vi "LS Data Loop.vi"(11 "FPGA Ref":T1) -> ()   [LabVIEW 2019]
uses:
  Controls/FPGA_Reference.ctl
  <vilib>/Utility/error.llb/Error Cluster From Error Code.vi
  <vilib>/rvi/errors/niLvFpgaAdjustHostInterfaceError.vi
  <vilib>/rvi/interface/nirviMethod/nirviMethod.xnode
  FPGA Bitfiles/LS_Durability_FPGA_9627.lvbitx
  <vilib>/rvi/interface/nirviReadWriteControl/nirviReadWriteControl.xnode
  <vilib>/rvi/errors/niLvFpgaMergeErrorWithErrorCode.vi
  <vilib>/FPGAPlugInAG/sbRIO-9627/niLvFpga_ReadFifo_sbRIO-9627.vi
  NiFpgaLv.dll
panel:
  out "FIFO loops":i32
  in  "LoopWait(ms)":u32=100
  in  "Sections":i32=100
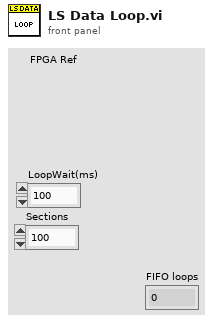
[diagram p1: front panel]
types:
  T1 = typedef "FPGA_Reference.ctl" = refnum<k20>
  T2 = cluster{"FPGA Ref":T1, "Time":dbl, "PtsTaken":i32, "Pts/File":i32, "10AveWait":u32, "Stored Filepath":path, "FileIndex":i32, "FilesUsed":i32, "Day":i32, "Anomaly Path":path}
  T3 = enum16{"Read", "Engine Writes", "Main Writes", "Write Anomalies", "Write Init Data"}
  T4 = enum16{"open", "replace", "create", "open or create", "replace or create", "replace or create with confirmation"}
  T5 = typedef "LS Data.ctl" = cluster{"Total Cycles":u32[], "Steps":u32[], "Anomalies Total":i32[], "Cycles":u32[], "Anomalies/Cycle":i32[], "Anomalies (Last Cycle)":i32[], "Opens":i32[]}
  T6 = cluster{"Running?":bool, "Profile Record":bool, "RecordInterval":i32, "RecordDuration":i32, "RecordFreq":i32, "Data Filepath":path, "Hr Record":bool, "Serial Numbers":string[]}
  T7 = typedef "LVDateTimeRec.ctl" = cluster{"fractional second":dbl, "second":i32, "minute":i32, "hour":i32, "day of month":i32, "month":i32, "year":i32, "day of week":i32, "day of year":i32, "DST":i32}
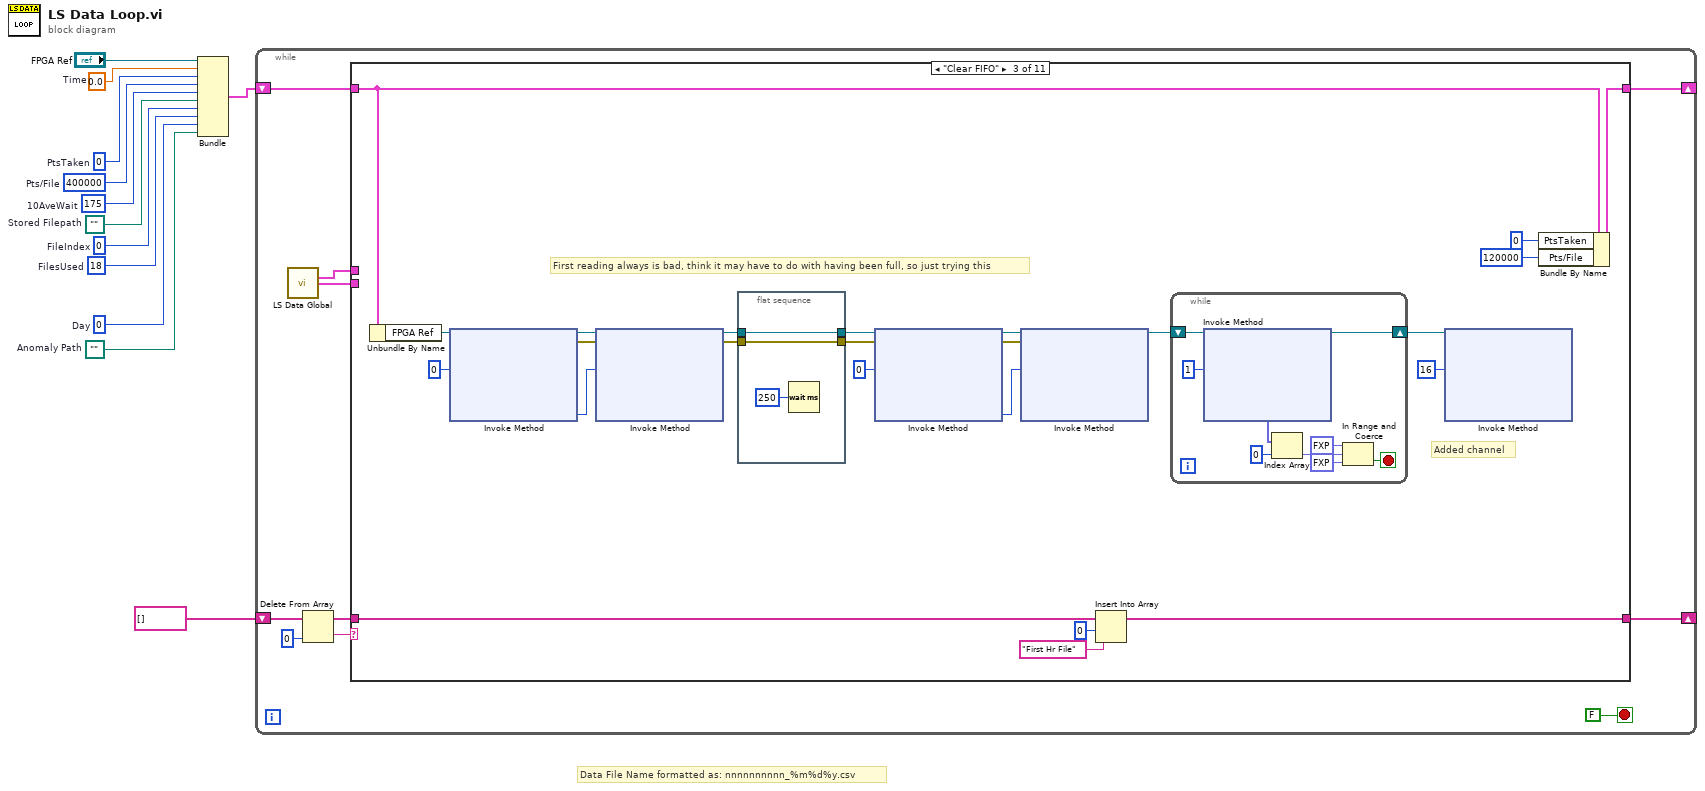
[diagram p0: block diagram]
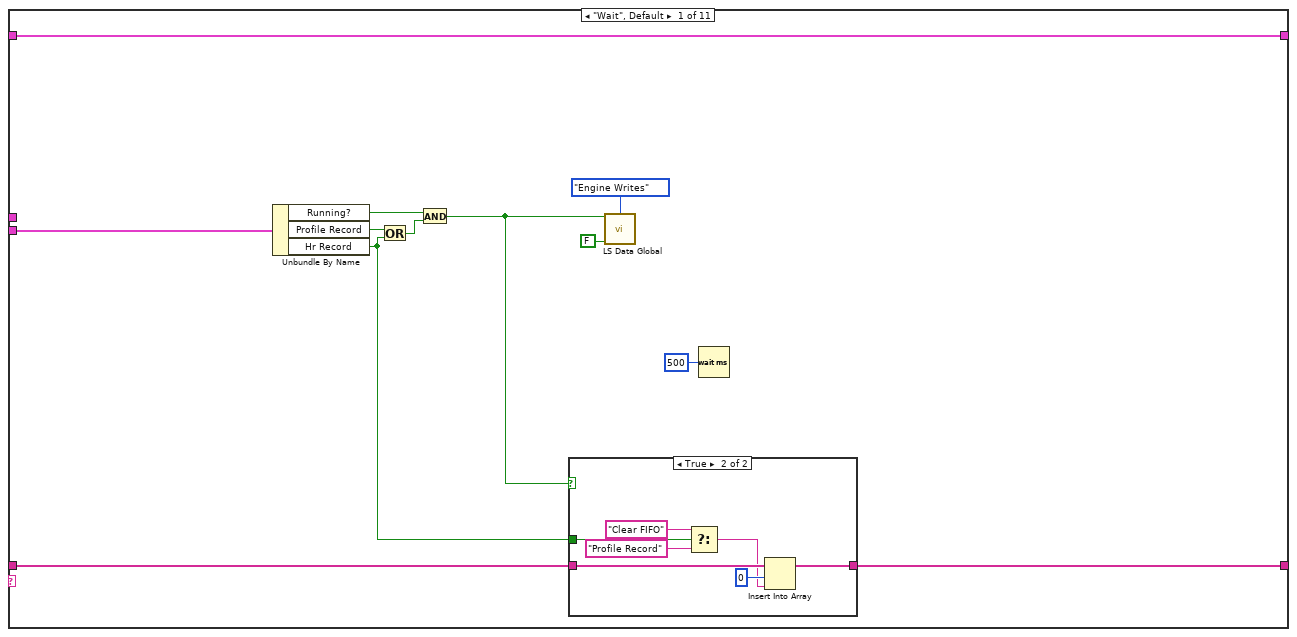
[diagram p2: hidden frame]
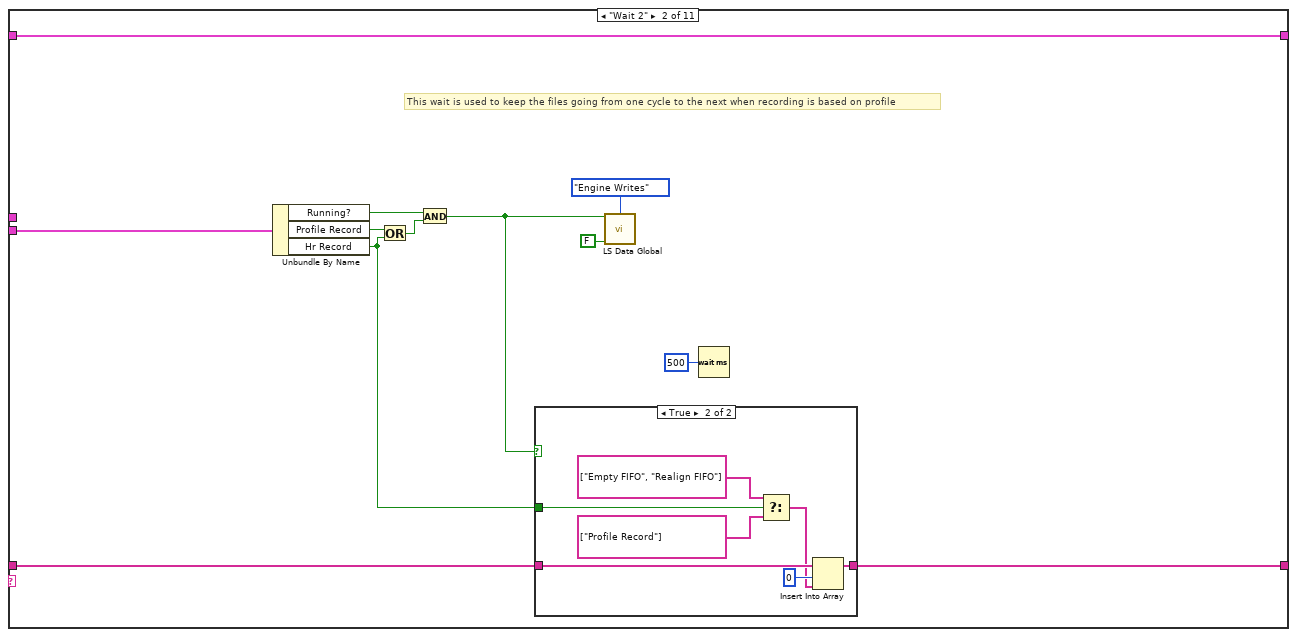
[diagram p4: hidden frame]
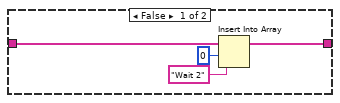
[diagram p5: hidden frame]
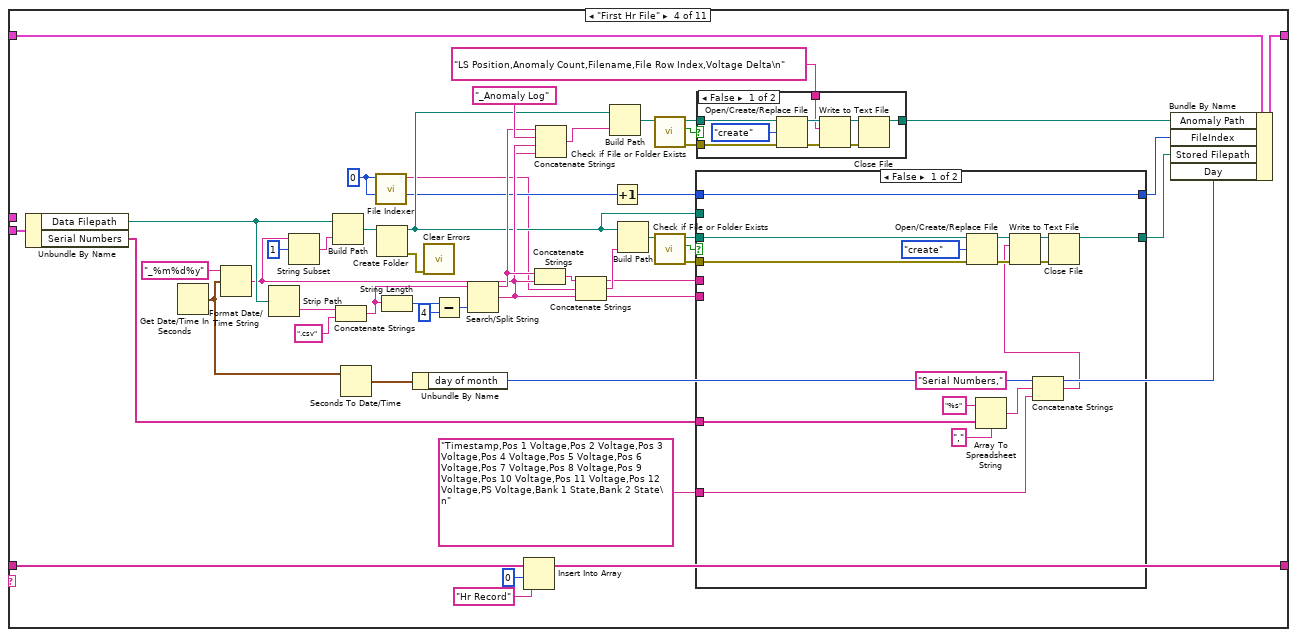
[diagram p6: hidden frame]
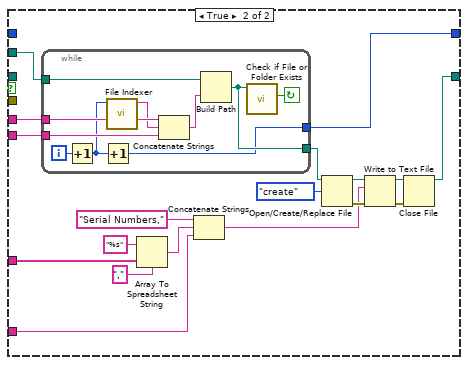
[diagram p8: hidden frame]
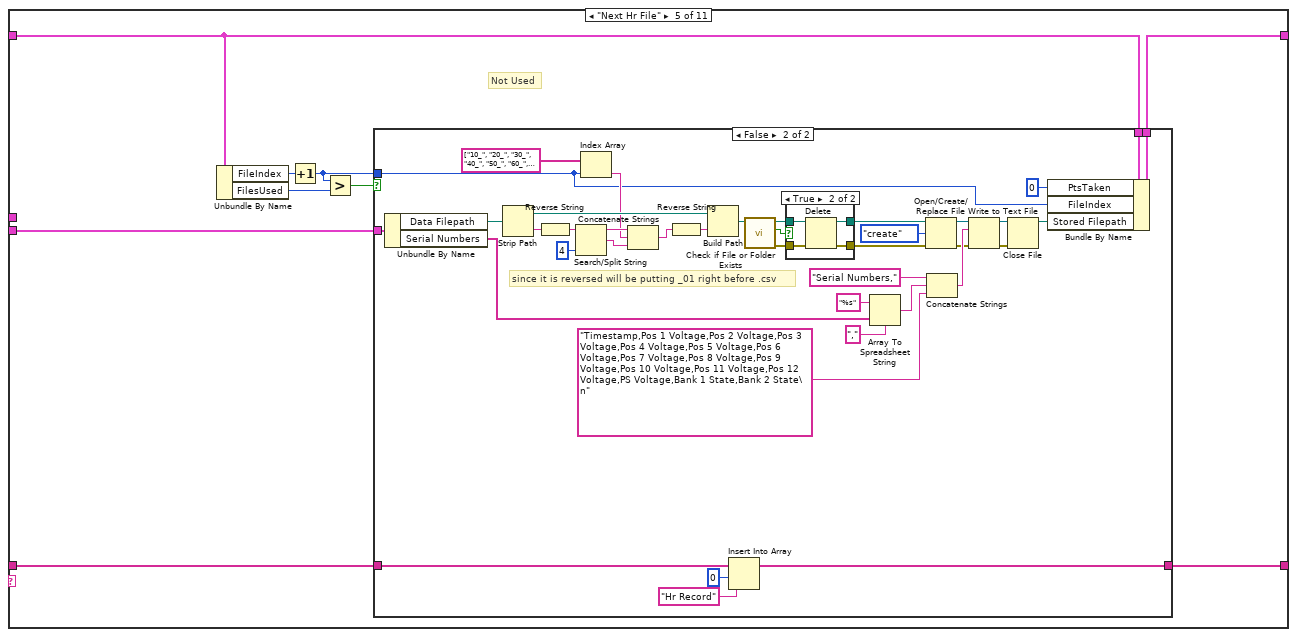
[diagram p9: hidden frame]
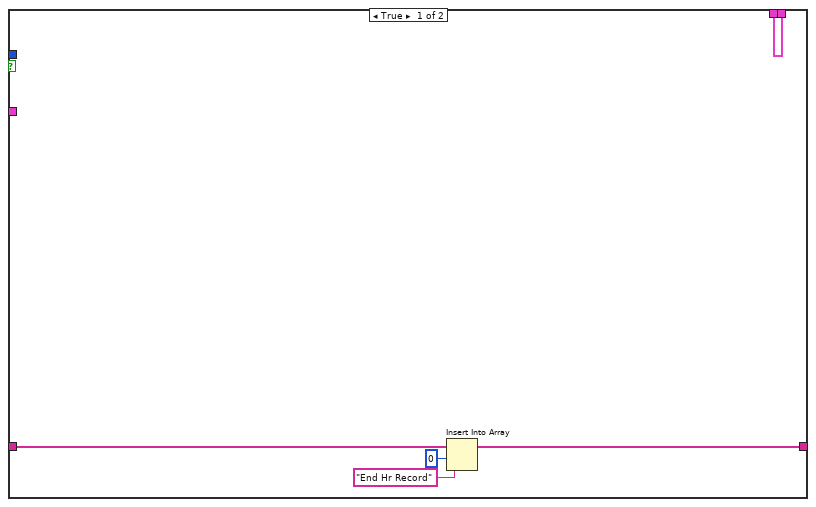
[diagram p10: hidden frame]
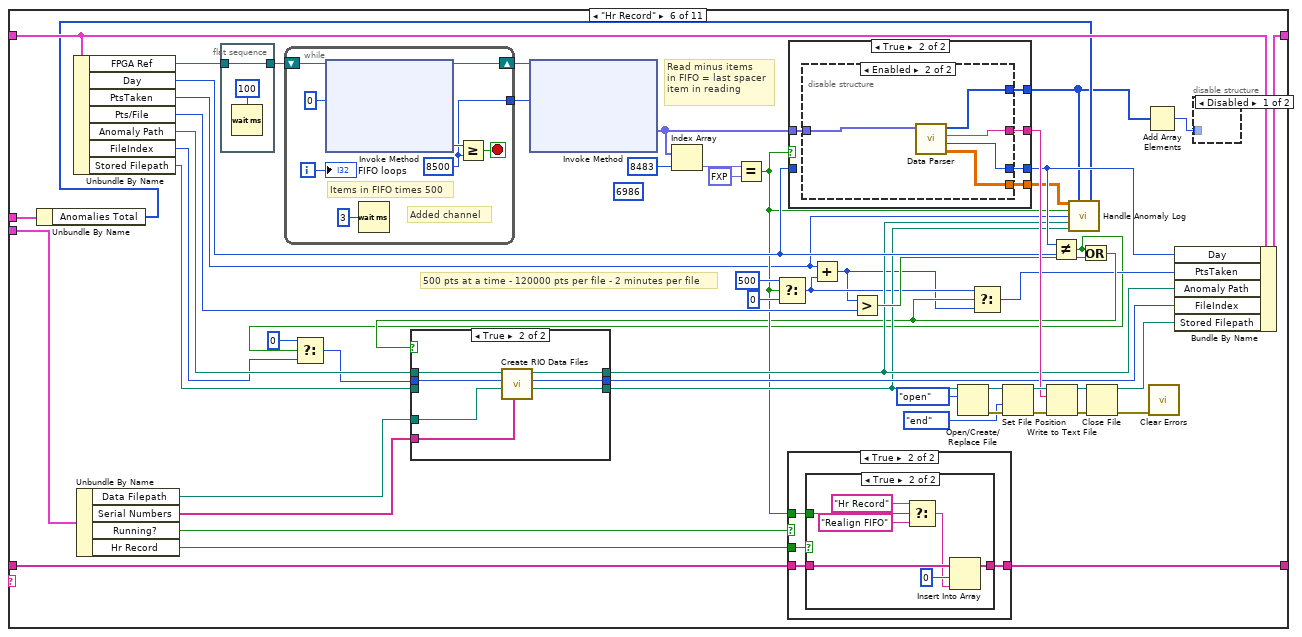
[diagram p12: hidden frame]
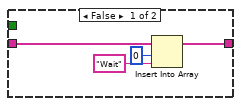
[diagram p14: hidden frame]
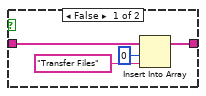
[diagram p15: hidden frame]
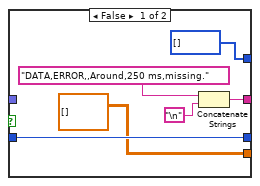
[diagram p17: hidden frame]
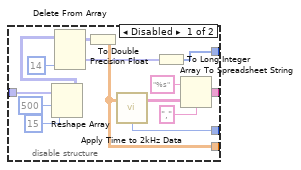
[diagram p18: hidden frame]
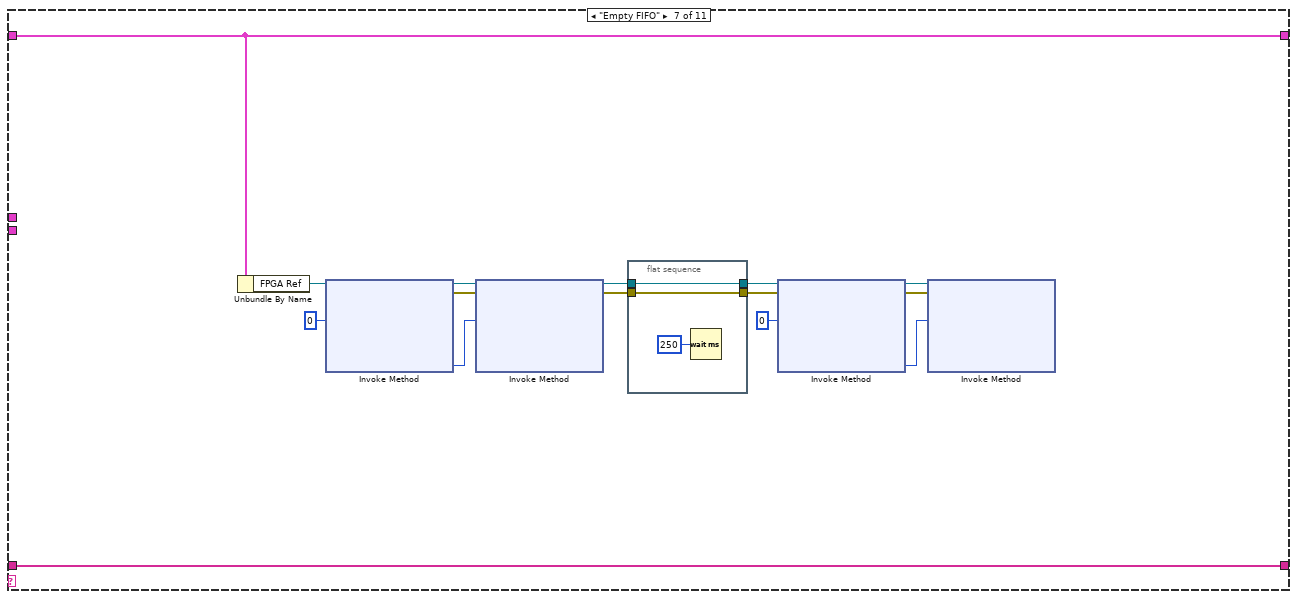
[diagram p19: hidden frame]
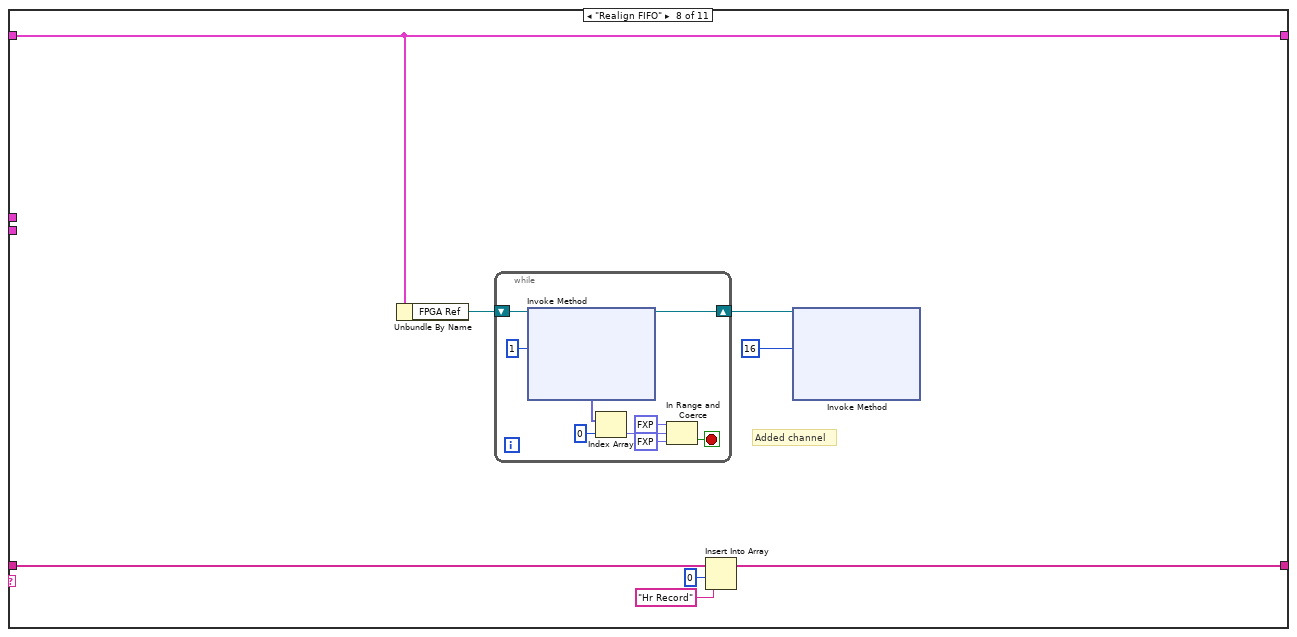
[diagram p20: hidden frame]
diagram:
  w1 = path ""  # Anomaly Path
  w2 = 0  # Day
  w3 = 18  # FilesUsed
  w4 = 0  # FileIndex
  w5 = path ""  # Stored Filepath
  w6 = u32 175  # 10AveWait
  w7 = 400000  # Pts/File
  w8 = 0  # PtsTaken
  w11 = 0.0  # Time
  # "Data File Name formatted as: nnnnnnnnnn_%m%d%y.csv"
  n1 = Bundle("FPGA Ref"="FPGA Ref", "Time"=w11, "PtsTaken"=w8, "Pts/File"=w7, "10AveWait"=w6, "Stored Filepath"=w5, "FileIndex"=w4, "FilesUsed"=w3, "Day"=w2, "Anomaly Path"=w1) -> (w10:T2)  [unwired: 1 in]
  n2 = while {
    shift-right: [w20] -> _
    shift-left: w10 -> [w21]
    shift-right: [w17] -> _
    shift-left: string[] [] -> [w19]
    stop <- FALSE stop-if-true
    n3 = call "LS Data Global.vi"() -> ("Initial LS Data Out"=w13:T5, "LS Cluster Out"=w18:T6)  [unwired: 12 in, 2 out]
    n4 = Delete From Array(array=w19, index=0) -> (deleted portion=w15:string, array with subset deleted=w14:string[])  [unwired: 1 in]
    n5 = case shown="\"Clear FIFO\"" w15 {
      tunnel: w14 -> [w31 w51 w85 w146 w203 w277 w398 w404 w428 w437 w440]
      tunnel: [w30 w50 w83 w145 w209 w276 w398 w403 w427 w436 w439] -> w17
      tunnel: w18 -> [w32 w52 _ w148 w211 w315 _ _ _ _ w441]
      tunnel: w21 -> [w29 w49 w81 w142 w208 w298 w399 w407 w424 w438 w443]
      tunnel: [w29 w49 w80 w147 w210 w297 w399 w407 w424 w438 w442] -> w20
      tunnel: w13 -> [_ _ _ _ _ w265 _ _ _ _ _]
      frame "Wait", Default {
        n6 = Unbundle By Name(w32) -> ("Running?"=w33:bool, "Profile Record"=w28:bool, "Hr Record"=w26:bool)
        n7 = Or(x=w28, y=w26) -> (x .or. y?=w27:bool)
        n8 = And(x=w33, y=w27) -> (x .and. y?=w25:bool)
        n9 = case shown="True" w25 {
          tunnel: w31 -> [w35 w42]
          tunnel: [w35 w41] -> w30
          tunnel: w26 -> [_ w39]
          frame False {
          }
          frame True {
            n10 = Select(t="Clear FIFO" ("new element/subarray"), s=w39, f="Profile Record" ("new element/subarray")) -> (s? t:f=w37:string)
            n11 = Insert Into Array(array=w42, index=0, new element=w37) -> (w41:string[])
          }
        }
        n12 = call "LS Data Global.vi"("Recording In"=w25, "Mode"=T3."Engine Writes", "Transferring In"=FALSE) -> ()  [unwired: 9 in, 4 out]
        n13 = Wait (ms)(milliseconds to wait=u32 500) -> ()  [unwired: 1 out]
      }
      frame "Wait 2" {
        # "This wait is used to keep the files going from one cycle to the next when recording is based on profile"
        n14 = Unbundle By Name(w52) -> ("Running?"=w53:bool, "Profile Record"=w48:bool, "Hr Record"=w46:bool)
        n15 = Or(x=w48, y=w46) -> (x .or. y?=w47:bool)
        n16 = And(x=w53, y=w47) -> (x .and. y?=w45:bool)
        n17 = case shown="True" w45 {
          tunnel: w51 -> [w58 w65]
          tunnel: [w57 w64] -> w50
          tunnel: w46 -> [_ w62]
          frame False {
            n18 = Insert Into Array(array=w58, index=0, new element="Wait 2" ("new element/subarray")) -> (w57:string[])
          }
          frame True {
            n19 = Select(t=string[] ["Empty FIFO", "Realign FIFO"], s=w62, f=string[] ["Profile Record"]) -> (s? t:f=w61:string[])
            n20 = Insert Into Array(array=w65, index=0, new element=w61) -> (w64:string[])
          }
        }
        n21 = call "LS Data Global.vi"("Recording In"=w45, "Mode"=T3."Engine Writes", "Transferring In"=FALSE) -> ()  [unwired: 9 in, 4 out]
        n22 = Wait (ms)(milliseconds to wait=u32 500) -> ()  [unwired: 1 out]
      }
      frame "Clear FIFO" {
        # "First reading always is bad, think it may have to do with having been full, so just trying this"
        # "Added channel"
        n23 = Unbundle By Name(w81) -> ("FPGA Ref"=w66:T1)
        n24 = xnode "Invoke Method"("FPGA VI Reference In"=w66, "Number of Elements"=u32 0) -> ("FPGA VI Reference Out"=w89:T1, "error out"=w88:errorcluster, "Elements Remaining"=w86:u32)  [unwired: 2 in, 1 out]
        n25 = xnode "Invoke Method"("FPGA VI Reference In"=w89, "error in"=w88, "Number of Elements"=w86) -> ("FPGA VI Reference Out"=w70:T1, "error out"=w69:errorcluster)  [unwired: 1 in, 2 out]
        n26 = flat-sequence {
          tunnel: w70 -> [w92]
          tunnel: w69 -> [w91]
          tunnel: [w92] -> w68
          tunnel: [w91] -> w67
          frame #0 {
            n27 = Wait (ms)(milliseconds to wait=u32 250) -> ()  [unwired: 1 out]
          }
        }
        n28 = xnode "Invoke Method"("FPGA VI Reference In"=w68, "error in"=w67, "Number of Elements"=u32 0) -> ("FPGA VI Reference Out"=w72:T1, "error out"=w73:errorcluster, "Elements Remaining"=w75:u32)  [unwired: 1 in, 1 out]
        n29 = xnode "Invoke Method"("FPGA VI Reference In"=w72, "error in"=w73, "Number of Elements"=w75) -> ("FPGA VI Reference Out"=w71:T1)  [unwired: 1 in, 3 out]
        n30 = Insert Into Array(array=w85, index=0, new element="First Hr File" ("new element/subarray")) -> (w83:string[])
        n31 = while {
          shift-right: [w100] -> w76
          shift-left: w71 -> [w101]
          stop <- w93 stop-if-true
          n32 = xnode "Invoke Method"("FPGA VI Reference In"=w101, "Number of Elements"=u32 1) -> ("FPGA VI Reference Out"=w100:T1, "Data"=w98:fxp<+/-,22,11>[])  [unwired: 2 in, 2 out]
          n33 = Index Array(array=w98, index=0) -> (element=w96:fxp<+/-,22,11>)
          n34 = In Range and Coerce(upper limit=fxp<+/-,18,5> -14.0, x=w96, lower limit=fxp<+/-,18,5> -15.0) -> (In Range?=w93:bool)  [unwired: 1 out]
        }
        n35 = xnode "Invoke Method"("FPGA VI Reference In"=w76, "Number of Elements"=u32 16) -> ()  [unwired: 2 in, 4 out]
        n36 = Bundle By Name(cluster=w81, "PtsTaken"=0, "Pts/File"=120000 ("PtsNeeded")) -> (w80:T2)
      }
      frame "First Hr File" {
        w104 = 0
        n37 = Unbundle By Name(w148) -> ("Data Filepath"=w127:path, "Serial Numbers"=w116:string[])
        n38 = Get Date/Time In Seconds() -> (seconds since 1Jan1904=w106:timestamp)
        n39 = Format Date/Time String(time format string (%c)="_%m%d%y", seconds (now)=w106) -> (date/time string=w112:string)  [unwired: 1 in]
        n40 = Strip Path(path=w127) -> (name=w139:string)  [unwired: 1 out]
        n41 = String Subset(string=w112, offset (0)=1) -> (substring=w137:string)  [unwired: 1 in]
        n42 = Build Path(base path=w127, name or relative path=w137) -> (appended path=w125:path)
        n43 = Concatenate Strings(w139, ".csv" ("string")) -> (w141:string)
        n44 = Seconds To Date/Time(time stamp (now)=w106) -> (date time rec=w107:T7)  [unwired: 1 in]
        n45 = call "File Indexer.vi"("File Index In"=w104) -> ("File Indicator Out"=w103:string)  [unwired: 10 in]
        n46 = Create Folder(path (use dialog)=w125) -> (created path=w108:path, error out=w126:errorcluster)  [unwired: 2 in, 1 out]
        n47 = String Length(string=w141) -> (length=w133:i32)
        n48 = Unbundle By Name(w107) -> ("day of month"=w105:i32)
        n49 = call <vilib>:"Clear Errors.vi"("error in (no error)"=w126) -> ()  [unwired: 5 in, 2 out]
        n50 = Subtract(x=w133, y=4) -> (x-y=w135:i32)
        n51 = Search/Split String(string=w141, offset (0)=w135) -> (substring before match=w113:string, match + rest of string=w109:string)  [unwired: 1 in, 1 out]
        n52 = Insert Into Array(array=w146, index=0, new element="Hr Record" ("new element/subarray")) -> (w145:string[])
        n53 = Concatenate Strings(w113, w112) -> (w110:string)
        n54 = Concatenate Strings(w113, "_Anomaly Log" ("string"), w112, w109) -> (w123:string)
        n55 = Concatenate Strings(w110, w103, w109) -> (w111:string)
        n56 = Build Path(base path=w108, name or relative path=w123) -> (appended path=w121:path)
        n57 = Increment(x=w104) -> (x+1=w115:i32)
        n58 = Build Path(base path=w108, name or relative path=w111) -> (appended path=w132:path)
        n59 = call <vilib>:"Check if File or Folder Exists.vi"("path"=w121) -> ("error out"=w118:errorcluster, "file or folder exists?"=w120:bool, "dup path"=w119:path)  [unwired: 8 in]
        n60 = call <vilib>:"Check if File or Folder Exists.vi"("path"=w132) -> ("error out"=w129:errorcluster, "file or folder exists?"=w131:bool, "dup path"=w130:path)  [unwired: 8 in]
        n61 = case shown="False" w131 {
          tunnel: w130 -> [w169 _]
          tunnel: [w168 w177] -> w124
          tunnel: w129 -> [w167 _]
          tunnel: w116 -> [w162 w184]
          tunnel: w115 -> [w160 _]
          tunnel: [w160 w189] -> w114
          tunnel: w110 -> [_ w191]
          tunnel: w109 -> [_ w190]
          tunnel: w108 -> [_ w192]
          tunnel: "Timestamp,Pos 1 Voltage,Pos 2 Voltage,Pos 3 Voltage,Pos 4 Voltage,Pos 5 Voltage,Pos 6 Voltage,Pos 7 Voltage,Pos 8 Voltage,Pos 9 Voltage,Pos 10 Voltage,Pos 11 Voltage,Pos 12 Voltage,PS Voltage,Bank 1 State,Bank 2 State\n" -> [w159 w175]
          frame False {
            n62 = Open/Create/Replace File(file path (use dialog)=w169, error in=w167, operation (0:open)=T4."create") -> (refnum out=w171:refnum<file>, error out=w173:errorcluster)  [unwired: 3 in, 1 out]
            n63 = Array To Spreadsheet String(delimiter (Tab)=",", array=w162, 3:"%s" ("format string")) -> (spreadsheet string=w163:string)
            n64 = Concatenate Strings("Serial Numbers," ("string"), w163, w159) -> (w161:string)
            n65 = Write to Text File(file (use dialog)=w171, text=w161, error in=w173) -> (refnum out=w170:refnum<file>, error out=w172:errorcluster)  [unwired: 1 in, 1 out]
            n66 = Close File(refnum=w170, error in=w172) -> (path=w168:path)  [unwired: 1 out]
          }
          frame True {
            n67 = while {
              tunnel: w192 -> [w202]
              tunnel: w191 -> [w201]
              tunnel: w190 -> [w200]
              tunnel: [w197] -> w178
              tunnel: [w195] -> w189
              i -> [w196]
              stop <- w198 continue-if-true
              n68 = Increment(x=w196) -> (x+1=w194:i32)
              n69 = Increment(x=w194) -> (x+1=w195:i32)
              n70 = call "File Indexer.vi"("File Index In"=w194) -> ("File Indicator Out"=w193:string)  [unwired: 10 in]
              n71 = Concatenate Strings(w201, w193, w200) -> (w199:string)
              n72 = Build Path(base path=w202, name or relative path=w199) -> (appended path=w197:path)
              n73 = call <vilib>:"Check if File or Folder Exists.vi"("path"=w197) -> ("file or folder exists?"=w198:bool)  [unwired: 8 in, 2 out]
            }
            n74 = Array To Spreadsheet String(delimiter (Tab)=",", array=w184, 3:"%s" ("format string")) -> (spreadsheet string=w185:string)
            n75 = Concatenate Strings("Serial Numbers," ("string"), w185, w175) -> (w176:string)
            n76 = Open/Create/Replace File(file path (use dialog)=w178, operation (0:open)=T4."create") -> (refnum out=w180:refnum<file>, error out=w182:errorcluster)  [unwired: 4 in, 1 out]
            n77 = Write to Text File(file (use dialog)=w180, text=w176, error in=w182) -> (refnum out=w179:refnum<file>, error out=w181:errorcluster)  [unwired: 1 in, 1 out]
            n78 = Close File(refnum=w179, error in=w181) -> (path=w177:path)  [unwired: 1 out]
          }
        }
        n79 = case shown="False" w120 {
          tunnel: w119 -> [w151 w158]
          tunnel: [w152 w158] -> w128
          tunnel: w118 -> [w150 _]
          tunnel: "LS Position,Anomaly Count,Filename,File Row Index,Voltage Delta\n" -> [w149 _]
          frame False {
            n80 = Open/Create/Replace File(file path (use dialog)=w151, error in=w150, operation (0:open)=T4."create") -> (refnum out=w154:refnum<file>, error out=w156:errorcluster)  [unwired: 3 in, 1 out]
            n81 = Write to Text File(file (use dialog)=w154, text=w149, error in=w156) -> (refnum out=w153:refnum<file>, error out=w155:errorcluster)  [unwired: 1 in, 1 out]
            n82 = Close File(refnum=w153, error in=w155) -> (path=w152:path)  [unwired: 1 out]
          }
          frame True {
          }
        }
        n83 = Bundle By Name(cluster=w142, "Anomaly Path"=w128, "FileIndex"=w114, "Stored Filepath"=w124, "Day"=w105) -> (w147:T2)
      }
      frame "Next Hr File" {
        # "Not Used"
        n84 = Unbundle By Name(w208) -> ("FileIndex"=w207:i32, "FilesUsed"=w206:i32)
        n85 = Increment(x=w207) -> (x+1=w205:i32)
        n86 = Greater?(x=w205, y=w206) -> (0:w204:bool)
        n87 = case shown="False" w204 {
          tunnel: w211 -> [_ w255]
          tunnel: [w216 w254] -> w210
          tunnel: [w214 w243] -> w209
          tunnel: w208 -> [w216 w222]
          tunnel: w205 -> [_ w220]
          tunnel: w203 -> [w215 w244]
          frame True {
            n88 = Insert Into Array(array=w215, index=0, new element="End Hr Record" ("new element/subarray")) -> (w214:string[])
          }
          frame False {
            # "since it is reversed will be putting _01 right before .csv"
            n89 = Unbundle By Name(w255) -> ("Data Filepath"=w253:path, "Serial Numbers"=w223:string[])
            n90 = Strip Path(path=w253) -> (stripped path=w252:path, name=w251:string)
            n91 = Reverse String(1:w251) -> (0:w249:string)
            n92 = Search/Split String(string=w249, offset (0)=4) -> (substring before match=w247:string, match + rest of string=w245:string)  [unwired: 1 in, 1 out]
            n93 = Index Array(array=string[] ["10_", "20_", "30_", "40_", "50_", "60_", "70_", "80_", "90_", "01_", "11_", "21_", "31_", "41_", "51_", "61_", "71_", "81_", "91_", "02_", "12_", "22_", "32_", "42_", "52_", "62_", "72_", "82_", "92_", "03_", "13_", "23_", "33_", "43_", "53_", "63_", "73_", "83_", "93_", "04_", "14_", "24_", "34_", "44_", "54_", "64_", "74_", "84_", "94_", "05_", "15_", "25_", "35_", "45_", "55_", "65_", "75_", "85_", "95_", "06_", "16_", "26_", "36_", "46_", "56_", "66_", "76_", "86_", "96_", "07_", "17_", "27_", "37_", "47_", "57_", "67_", "77_", "87_", "97_", "08_", "18_", "28_", "38_", "48_", "58_", "68_", "78_", "88_", "98_", "09_", "19_", "29_", "39_", "49_", "59_", "69_", "79_", "89_", "99_"] ("Array 2"), index=w220) -> (element=w221:string)
            n94 = Concatenate Strings(w247, w221, w245) -> (w246:string)
            n95 = Reverse String(1:w246) -> (0:w250:string)
            n96 = Build Path(base path=w252, name or relative path=w250) -> (appended path=w240:path)
            n97 = Insert Into Array(array=w244, index=0, new element="Hr Record" ("new element/subarray")) -> (w243:string[])
            n98 = call <vilib>:"Check if File or Folder Exists.vi"("path"=w240) -> ("error out"=w225:errorcluster, "file or folder exists?"=w239:bool, "dup path"=w238:path)  [unwired: 8 in]
            n99 = case shown="True" w239 {
              tunnel: w238 -> [w257 w261]
              tunnel: [w257 w260] -> w227
              tunnel: w225 -> [w256 w259]
              tunnel: [w256 w258] -> w224
              frame False {
              }
              frame True {
                n100 = Delete(path (use dialog)=w261, error in=w259) -> (deleted path=w260:path, error out=w258:errorcluster)  [unwired: 3 in, 1 out]
              }
            }
            n101 = Array To Spreadsheet String(delimiter (Tab)=",", array=w223, 3:"%s" ("format string")) -> (spreadsheet string=w237:string)
            n102 = Open/Create/Replace File(file path (use dialog)=w227, error in=w224, operation (0:open)=T4."create") -> (refnum out=w231:refnum<file>, error out=w229:errorcluster)  [unwired: 3 in, 1 out]
            n103 = Concatenate Strings("Serial Numbers," ("string"), w237, "Timestamp,Pos 1 Voltage,Pos 2 Voltage,Pos 3 Voltage,Pos 4 Voltage,Pos 5 Voltage,Pos 6 Voltage,Pos 7 Voltage,Pos 8 Voltage,Pos 9 Voltage,Pos 10 Voltage,Pos 11 Voltage,Pos 12 Voltage,PS Voltage,Bank 1 State,Bank 2 State\n") -> (w234:string)
            n104 = Write to Text File(file (use dialog)=w231, text=w234, error in=w229) -> (refnum out=w232:refnum<file>, error out=w230:errorcluster)  [unwired: 1 in, 1 out]
            n105 = Close File(refnum=w232, error in=w230) -> (path=w226:path)  [unwired: 1 out]
            n106 = Bundle By Name(cluster=w222, "PtsTaken"=0, "FileIndex"=w220, "Stored Filepath"=w226) -> (w254:T2)
          }
        }
      }
      frame "Hr Record" {
        (unwired) 6986 ("index")
        # "Read minus items\nin FIFO = last spacer\nitem in reading"
        # "500 pts at a time - 120000 pts per file - 2 minutes per file"
        n107 = Unbundle By Name(w265) -> ("Anomalies Total"=w264:i32[])
        n108 = Unbundle By Name(w298) -> ("FPGA Ref"=w303:T1, "Day"=w290:i32, "PtsTaken"=w274:i32, "Pts/File"=w296:i32, "Anomaly Path"=w288:path, "FileIndex"=w268:i32, "Stored Filepath"=w287:path)
        n109 = Unbundle By Name(w315) -> ("Data Filepath"=w275:path, "Serial Numbers"=w284:string[], "Running?"=w279:bool, "Hr Record"=w278:bool)
        n110 = flat-sequence {
          tunnel: w303 -> [w376]
          tunnel: [w376] -> w302
          frame #0 {
            n111 = Wait (ms)(milliseconds to wait=u32 100) -> ()  [unwired: 1 out]
          }
        }
        n112 = while {
          tunnel: [w382] -> w314
          shift-right: [w379] -> w313
          shift-left: w302 -> [w380]
          i -> [w378]
          stop <- w381 stop-if-true
          w382 = u32 8500 ("y")
          # "Added channel"
          # "Items in FIFO times 500"
          n113 = xnode "Invoke Method"("FPGA VI Reference In"=w380, "Number of Elements"=u32 0) -> ("FPGA VI Reference Out"=w379:T1, "Elements Remaining"=w383:u32)  [unwired: 2 in, 2 out]
          n114 = Wait (ms)(milliseconds to wait=u32 3) -> ()  [unwired: 1 out]
          n115 = Greater Or Equal?(x=w383, y=w382) -> (x >= y?=w381:bool)
          "FIFO loops" <- w378
        }
        n116 = xnode "Invoke Method"("FPGA VI Reference In"=w313, "Number of Elements"=w314) -> ("Data"=w295:fxp<+/-,22,11>[])  [unwired: 2 in, 3 out]
        n117 = Index Array(array=w295, index=8483) -> (element=w294:fxp<+/-,22,11>)
        n118 = Equal?(x=w294, y=fxp<+/-,18,5> -15.0) -> (x = y?=w280:bool)
        n119 = Select(t=500 ("PtsTaken"), s=w280, f=0 ("PtsTaken")) -> (s? t:f=w272:i32)
        n120 = case shown="True" w279 {
          tunnel: w277 -> [w318 w323]
          tunnel: [w317 w322] -> w276
          tunnel: w280 -> [_ w320]
          tunnel: w278 -> [_ w321]
          frame False {
            n121 = Insert Into Array(array=w318, index=0, new element="Wait") -> (w317:string[])
          }
          frame True {
            n122 = case shown="True" w321 {
              tunnel: w323 -> [w327 w334]
              tunnel: [w326 w333] -> w322
              tunnel: w320 -> [_ w331]
              frame False {
                n123 = Insert Into Array(array=w327, index=0, new element="Transfer Files") -> (w326:string[])
              }
              frame True {
                n124 = Select(t="Hr Record", s=w331, f="Realign FIFO" ("new element/subarray")) -> (s? t:f=w329:string)
                n125 = Insert Into Array(array=w334, index=0, new element=w329) -> (w333:string[])
              }
            }
          }
        }
        n126 = case shown="True" w280 {
          tunnel: [w348 w355] -> w292
          tunnel: w295 -> [_ w353]
          tunnel: [w347 w354] -> w291
          tunnel: w290 -> [w347 _]
          tunnel: [dbl[][] [] w352] -> w283
          tunnel: [i32[] [] w351] -> w263
          frame False {
            n127 = Concatenate Strings("DATA,ERROR,,Around,250 ms,missing." ("string"), "\n") -> (w348:string)
          }
          frame True {
            n128 = disable-structure shown="Enabled" {
              disable-tunnel: [w365 w372] -> w355
              disable-tunnel: [w363 w371] -> w354
              disable-tunnel: w353 -> [w362 w374]
              disable-tunnel: [w358 w370] -> w352
              disable-tunnel: [w356 w373] -> w351
              frame Disabled {
                n129 = Reshape Array(w362, 500 ("dimension size"), 15 ("dimension size")) -> (w361:fxp<+/-,22,11>[][])
                n130 = Delete From Array(array=w361, index (col)=14 ("disabled index (col)")) -> (deleted portion=w357:fxp<+/-,22,11>[], array with subset deleted=w359:fxp<+/-,22,11>[][])  [unwired: 2 in]
                n131 = To Double Precision Float(number=w359) -> (double precision float=w358:dbl[][])
                n132 = call "Apply Time to 2kHz Data.vi"("Data In"=w358) -> ("Day"=w363:i32, "Data Out"=w364:string[][])  [unwired: 2 in]
                n133 = To Long Integer(number=w357) -> (32bit integer=w356:i32[])
                n134 = Array To Spreadsheet String(delimiter (Tab)=",", array=w364, 3:"%s" ("format string")) -> (spreadsheet string=w365:string)
              }
              frame Enabled {
                n135 = call "Data Parser.vi"("Raw Data"=w374) -> ("Data Out"=w370:dbl[][], "Day"=w371:i32, "CSV String"=w372:string, "Anomaly Array"=w373:i32[])  [unwired: 7 in]
              }
            }
          }
        }
        n136 = Add(x=w274, y=w272) -> (x+y=w271:i32)
        n137 = Greater?(x=w271, y=w296) -> (0:w289:bool)
        n138 = Not Equal?(x=w291, y=w290) -> (x != y?=w269:bool)
        n139 = Select(t=0, s=w269, f=w268) -> (s? t:f=w267:i32)
        n140 = Or(x=w269, y=w289) -> (x .or. y?=w273:bool)
        n141 = case shown="True" w273 {
          tunnel: w287 -> [w337 _]
          tunnel: [w337 w344] -> w281
          tunnel: w288 -> [w336 w343]
          tunnel: [w336 w342] -> w282
          tunnel: w267 -> [w335 w341]
          tunnel: [w335 w340] -> w285
          tunnel: w284 -> [_ w339]
          tunnel: w275 -> [_ w338]
          frame False {
          }
          frame True {
            n142 = call "Create RIO Data Files.vi"("Serial Numbers"=w339, "Base Filepath"=w338, "File Index In"=w341, "Anomaly Filepath In"=w343) -> ("Current Filepath"=w344:path, "File Index Out"=w340:i32, "Anomaly Filepath Out"=w342:path)  [unwired: 5 in]
          }
        }
        n143 = Open/Create/Replace File(file path (use dialog)=w281, operation (0:open)=T4."open") -> (refnum out=w308:refnum<file>, error out=w307:errorcluster)  [unwired: 4 in, 1 out]
        n144 = Select(t=w272, s=w273, f=w271) -> (s? t:f=w270:i32)
        n145 = Set File Position(refnum=w308, from (0:start)=enum16{"start", "end", "current"}."end", error in=w307) -> (refnum out=w305:refnum<file>, error out=w304:errorcluster)  [unwired: 1 in]
        n146 = Write to Text File(file (use dialog)=w305, text=w292, error in=w304) -> (refnum out=w311:refnum<file>, error out=w312:errorcluster)  [unwired: 1 in, 1 out]
        n147 = call "Handle Anomaly Log.vi"("Data"=w283, "FPGAnomalies"=w263, "Init Anomalies"=w264, "Enable"=w280, "RowCount In"=w274, "Anomaly Log Path"=w282, "Current Data Path"=w281) -> ()  [unwired: 9 in]
        n148 = Close File(refnum=w311, error in=w312) -> (path=w286:path, error out=w310:errorcluster)
        n149 = Add Array Elements(numeric array=w263) -> (sum=w262:i32)
        n150 = call <vilib>:"Clear Errors.vi"("error in (no error)"=w310) -> ()  [unwired: 5 in, 2 out]
        n151 = Bundle By Name(cluster=w298, "Day"=w291, "PtsTaken"=w270, "Anomaly Path"=w282, "FileIndex"=w285, "Stored Filepath"=w286) -> (w297:T2)
        n152 = disable-structure shown="Disabled" {
          disable-tunnel: w262 -> [_ _]
          frame Disabled {
          }
          frame Enabled {
          }
        }
      }
      frame "Empty FIFO" {
        n153 = Unbundle By Name(w399) -> ("FPGA Ref"=w397:T1)
        n154 = xnode "Invoke Method"("FPGA VI Reference In"=w397, "Number of Elements"=u32 0) -> ("FPGA VI Reference Out"=w396:T1, "error out"=w395:errorcluster, "Elements Remaining"=w393:u32)  [unwired: 2 in, 1 out]
        n155 = xnode "Invoke Method"("FPGA VI Reference In"=w396, "error in"=w395, "Number of Elements"=w393) -> ("FPGA VI Reference Out"=w388:T1, "error out"=w387:errorcluster)  [unwired: 1 in, 2 out]
        n156 = flat-sequence {
          tunnel: w388 -> [w402]
          tunnel: w387 -> [w401]
          tunnel: [w402] -> w386
          tunnel: [w401] -> w385
          frame #0 {
            n157 = Wait (ms)(milliseconds to wait=u32 250) -> ()  [unwired: 1 out]
          }
        }
        n158 = xnode "Invoke Method"("FPGA VI Reference In"=w386, "error in"=w385, "Number of Elements"=u32 0) -> ("FPGA VI Reference Out"=w389:T1, "error out"=w390:errorcluster, "Elements Remaining"=w392:u32)  [unwired: 1 in, 1 out]
        n159 = xnode "Invoke Method"("FPGA VI Reference In"=w389, "error in"=w390, "Number of Elements"=w392) -> ()  [unwired: 1 in, 4 out]
      }
      frame "Realign FIFO" {
        # "Added channel"
        n160 = Unbundle By Name(w407) -> ("FPGA Ref"=w410:T1)
        n161 = while {
          shift-right: [w418] -> w408
          shift-left: w410 -> [w419]
          stop <- w411 stop-if-true
          n162 = xnode "Invoke Method"("FPGA VI Reference In"=w419, "Number of Elements"=u32 1) -> ("FPGA VI Reference Out"=w418:T1, "Data"=w416:fxp<+/-,22,11>[])  [unwired: 2 in, 2 out]
          n163 = Index Array(array=w416, index=0) -> (element=w414:fxp<+/-,22,11>)
          n164 = In Range and Coerce(upper limit=fxp<+/-,18,5> -14.0, x=w414, lower limit=fxp<+/-,18,5> -15.0) -> (In Range?=w411:bool)  [unwired: 1 out]
        }
        n165 = Insert Into Array(array=w404, index=0, new element="Hr Record" ("new element/subarray")) -> (w403:string[])
        n166 = xnode "Invoke Method"("FPGA VI Reference In"=w408, "Number of Elements"=u32 16) -> ()  [unwired: 2 in, 4 out]
      }
      frame "Transfer Files" {
        # "Not transferring the current data or anomaly file in case they are still to be written to"
        n167 = Unbundle By Name(w424) -> ("Stored Filepath"=w423:path, "Anomaly Path"=w422:path)
        n168 = Build Array(w423, w422) -> (w420:path[])
        n169 = flat-sequence {
          tunnel: [w430] -> w421
          tunnel: w420 -> [w430]
          tunnel: w421 -> [w433]
          frame #0 {
            n170 = call "LS Data Global.vi"("Recording In"=FALSE, "Mode"=T3."Engine Writes", "Transferring In"=TRUE) -> ()  [unwired: 9 in, 4 out]
          }
          frame #1 {
            n171 = call "WebDAV mass transfer.vi"("Prevented Files"=w433) -> ()  [unwired: 11 in]
          }
        }
        n172 = Insert Into Array(array=w428, index=0, new element="Wait 2" ("new element/subarray")) -> (w427:string[])
      }
      frame "End Hr Record" {
        n173 = Insert Into Array(array=w437, index=0, new element="Wait" ("new element/subarray")) -> (w436:string[])
      }
      frame "Profile Record" {
        n174 = disable-structure shown="Enabled" {
          disable-tunnel: w443 -> [w469 w563]
          disable-tunnel: [w468 w563] -> w442
          disable-tunnel: w441 -> [w467 _]
          disable-tunnel: w440 -> [w450 w562]
          disable-tunnel: [w449 w562] -> w439
          frame Disabled {
            n175 = Unbundle By Name(w469) -> ("FPGA Ref"=w461:T1, "Time"=w455:dbl)
            n176 = Unbundle By Name(w467) -> ("Running?"=w452:bool, "Profile Record"=w451:bool, "RecordDuration"=w464:i32, "RecordFreq"=w465:i32, "Data Filepath"=w466:path, "RecordInterval"=w453:i32)
            n177 = Get Date/Time In Seconds() -> (seconds since 1Jan1904=w463:timestamp)
            n178 = To Double Precision Float(number=w463) -> (double precision float=w456:dbl)
            n179 = Subtract(x=w456, y=w455) -> (x-y=w460:dbl)
            n180 = Subtract(x=w453, y=w460) -> (x-y=w454:dbl)
            n181 = Empty String/Path?(string/path=w466) -> (empty?=w458:bool)
            n182 = And(x=w452, y=w451) -> (x .and. y?=w447:bool)
            n183 = Less Or Equal To 0?(x=w454) -> (x <= 0?=w459:bool)
            n184 = Compound Arithmetic op=AND(invert w458, w459) -> (w457:bool)
            n185 = Select(t="Profile Record", s=w447, f="Wait") -> (s? t:f=w444:string)
            n186 = case shown="True" w457 {
              tunnel: w465 -> [_ w500]
              tunnel: w464 -> [_ w506]
              tunnel: w461 -> [_ w503]
              tunnel: w456 -> [_ w502]
              tunnel: [w478 w502] -> w462
              tunnel: w455 -> [w478 _]
              tunnel: w454 -> [w472 _]
              tunnel: w466 -> [_ w479]
              frame False {
                w477 = u32 500 ("milliseconds to wait")
                n187 = Multiply(x=1000.0 ("y"), y=w472) -> (x*y=w474:dbl)
                n188 = To Unsigned Long Integer(number=w474) -> (unsigned 32bit integer=w471:u32)
                n189 = Less?(x=w477, y=w471) -> (x < y?=w475:bool)
                n190 = Increment(x=w471) -> (x+1=w470:u32)
                n191 = Select(t=w477, s=w475, f=w470) -> (s? t:f=w476:u32)
                n192 = Wait (ms)(milliseconds to wait=w476) -> ()  [unwired: 1 out]
              }
              frame True {
                n193 = Divide(x=1000, y=w500) -> (x/y=w505:dbl)
                n194 = Multiply(x=w506, y=w500) -> (x*y=w493:i32)
                n195 = Round Toward -Infinity(1:w505) -> (0:w507:dbl)
                n196 = Subtract(x=w505, y=w507) -> (x-y=w499:dbl)
                n197 = To Unsigned Long Integer(number=w505) -> (unsigned 32bit integer=w504:u32)
                n198 = flat-sequence {
                  tunnel: w499 -> [w510]
                  tunnel: w503 -> [w511]
                  tunnel: w504 -> [w512]
                  tunnel: w493 -> [w513]
                  tunnel: [w513] -> w498
                  tunnel: [w512] -> w497
                  tunnel: [w511] -> w496
                  tunnel: [w510] -> w495
                  tunnel: [w509] -> w488
                  tunnel: [w508] -> w480
                  tunnel: w479 -> [w508]
                  tunnel: w498 -> [w516]
                  tunnel: w497 -> [w520]
                  tunnel: w496 -> [w519]
                  tunnel: w495 -> [w514]
                  tunnel: [w518] -> w494
                  tunnel: [w517] -> w489
                  tunnel: w488 -> [w517]
                  tunnel: [w516] -> w486
                  tunnel: [w515] -> w481
                  tunnel: w480 -> [w515]
                  tunnel: w494 -> [w537]
                  tunnel: [w537] -> w492
                  tunnel: [w536] -> w491
                  tunnel: [w535] -> w490
                  tunnel: w489 -> [w535]
                  tunnel: [w534] -> w487
                  tunnel: w486 -> [w534]
                  tunnel: [w533] -> w482
                  tunnel: w481 -> [w533]
                  tunnel: w492 -> [w553]
                  tunnel: w491 -> [w547]
                  tunnel: w490 -> [w546]
                  tunnel: w487 -> [w545]
                  tunnel: [w553] -> w485
                  tunnel: [w543] -> w484
                  tunnel: [w540] -> w483
                  tunnel: w482 -> [w540]
                  tunnel: w483 -> [w559]
                  tunnel: w484 -> [w560]
                  tunnel: w485 -> [w561]
                  frame #0 {
                    n199 = Get Date/Time In Seconds() -> (seconds since 1Jan1904=w509:timestamp)
                  }
                  frame #1 {
                    n200 = for {
                      N: w516 -> [_]
                      tunnel: w520 -> [w532]
                      shift-right: [w529] -> _
                      shift-left: w514 -> [w530]
                      tunnel: w514 -> [w528]
                      tunnel: w519 -> [w527]
                      tunnel: [w525] -> w518 mode=indexing
                      n201 = xnode "Read/Write Control"("FPGA VI Reference In"=w527) -> ("Analog Inputs"=w526:fxp<+/-,28,17>[])  [unwired: 1 in, 2 out]
                      n202 = Greater Or Equal?(x=w530, y=1.0) -> (x >= y?=w523:bool)
                      n203 = Boolean To (0,1)(Boolean=w523) -> (0, 1=w522:i16)
                      n204 = Add(x=w532, y=w522) -> (x+y=w531:u32)
                      n205 = Subtract(x=w530, y=w522) -> (x-y=w521:dbl)
                      n206 = Add(x=w521, y=w528) -> (x+y=w529:dbl)
                      n207 = Wait (ms)(milliseconds to wait=w531) -> ()  [unwired: 1 out]
                      n208 = To Double Precision Float(number=w526) -> (double precision float=w525:dbl[])
                    }
                  }
                  frame #2 {
                    n209 = Get Date/Time In Seconds() -> (seconds since 1Jan1904=w536:timestamp)
                  }
                  frame #3 {
                    w542 = 86400.0 ("y")
                    n210 = To Double Precision Float(number=w547) -> (double precision float=w541:dbl)
                    n211 = To Double Precision Float(number=w546) -> (double precision float=w538:dbl)
                    n212 = Decrement(x=w545) -> (x-1=w544:i32)
                    n213 = Subtract(x=w541, y=w538) -> (x-y=w539:dbl)
                    n214 = Divide(x=w539, y=w544) -> (x/y=w548:dbl)
                    n215 = Divide(x=w548, y=w542) -> (x/y=w552:dbl)
                    n216 = Divide(x=w538, y=w542) -> (x/y=w549:dbl)
                    n217 = Add(x=w549, y=1462.0) -> (x+y=w551:dbl)
                    n218 = for {
                      N: w545 -> [_]
                      shift-right: [w554] -> _
                      shift-left: w551 -> [w555]
                      tunnel: w552 -> [w556]
                      tunnel: [w555] -> w543 mode=indexing
                      n219 = Add(x=w556, y=w555) -> (x+y=w554:dbl)
                    }
                  }
                  frame #4 {
                    n220 = call "Format Data to Save.vi"("Sections"="Sections", "FilePath"=w559, "LoopBeginWait(ms)"="LoopWait(ms)", "Time"=w560, "Data"=w561) -> ()  [unwired: 7 in]
                  }
                }
              }
            }
            n221 = Insert Into Array(array=w450, index=0, new element=w444) -> (w449:string[])
            n222 = Bundle By Name(cluster=w469, "Time"=w462) -> (w468:T2)
          }
          frame Enabled {
          }
        }
      }
    }
  }
